vi "responseMSEARCH.vi"(1 "root":T1) -> (0 "ucastResponseMSG":string)   [LabVIEW 2010]
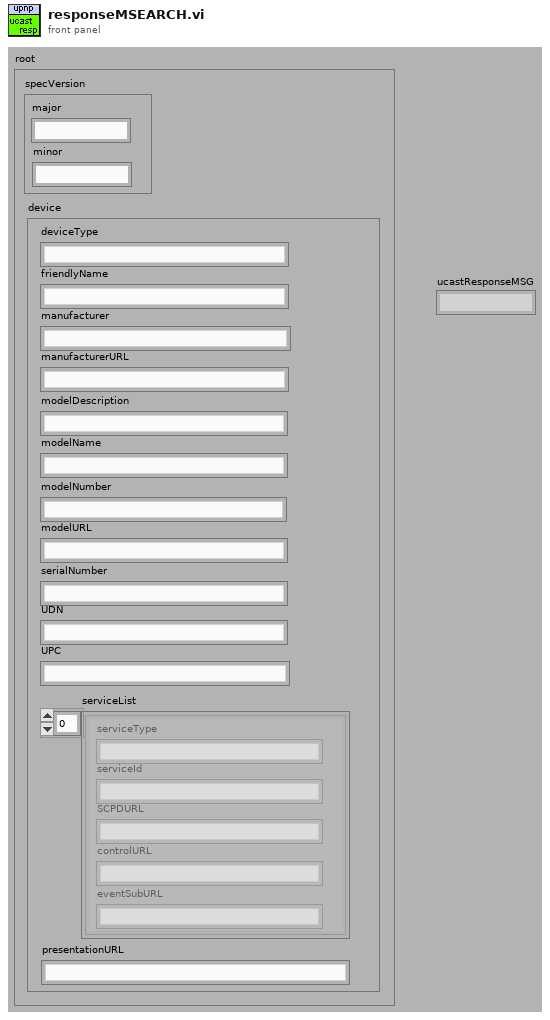
[diagram p1: front panel]
types:
  T1 = cluster{"specVersion":cluster{"major":string, "minor":string}, "device":cluster{"deviceType":string, "friendlyName":string, "manufacturer":string, "manufacturerURL":string, "modelDescription":string, "modelName":string, "modelNumber":string, "modelURL":string, "serialNumber":string, "UDN":string, "UPC":string, "serviceList":cluster{"serviceType":string, "serviceId":string, "SCPDURL":string, "controlURL":string, "eventSubURL":string}[], "presentationURL":string}}
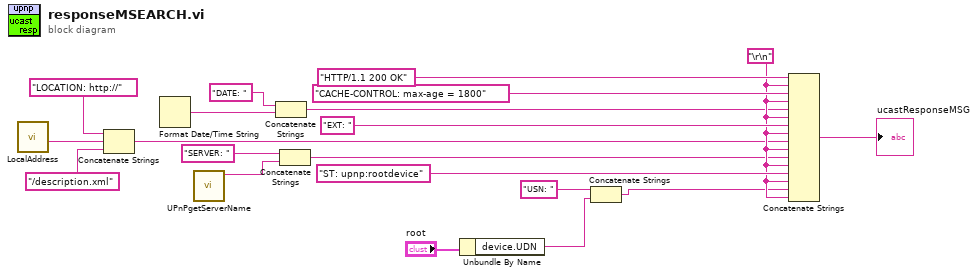
[diagram p0: block diagram]
diagram:
  w16 = "\r\n"
  n1 = call "LocalAddress.vi"() -> ("IP Address (xx.xx.xx.xx)"=w8:string)  [unwired: 11 out]
  n2 = Concatenate Strings("LOCATION: http://" ("string"), w8, "/description.xml" ("string")) -> (w5:string)
  n3 = Format Date/Time String() -> (date/time string=w13:string)  [unwired: 3 out]
  n4 = call "UPnPgetServerName.vi"() -> ("ServerName"=w9:string)  [unwired: 11 out]
  n5 = Concatenate Strings("DATE: " ("string"), w13) -> (w12:string)
  n6 = Concatenate Strings("SERVER: " ("string"), w9) -> (w11:string)
  n7 = Unbundle By Name("root") -> ("device.UDN"=w1:string)
  n8 = Concatenate Strings("USN: " ("string"), w1) -> (w3:string)
  n9 = Concatenate Strings("HTTP/1.1 200 OK" ("string"), w16, "CACHE-CONTROL: max-age = 1800" ("string"), w16, w12, w16, "EXT: " ("string"), w16, w5, w16, w11, w16, "ST: upnp:rootdevice" ("string"), w16, w3, w16) -> (→"ucastResponseMSG":string)
